vi "Command_ShootFromPose.vi"(0 "Startup":bool, 2 "Shooter_table":dbl[][](array[numeric]), 3 "Timeout":dbl) -> (11 "Reint":bool, 12 "turret_angle(deg)":dbl, 14 "Completed":bool, 15 "turret_state":T3=enum."No-Op", 16 "flywheel_state":T2, 17 "flywheel_speed(RPM)":dbl, 18 "cowl_state":T1=enum."No-Op", 19 "cowl_angle(deg)":dbl)   [LabVIEW 2020]
uses:
  Subsystems/Turret/Turret_States.ctl
  Subsystems/Flywheel/Flywheel_States.ctl
  Subsystems/Cowl/Cowl_States.ctl
  Auto Utilities/Command_Execution_State.ctl
  Globals/Sensor_Values.vi
  Systems/Shooter/Determiner/Shooter_Globals.vi
  Globals/Drive_Globals.vi
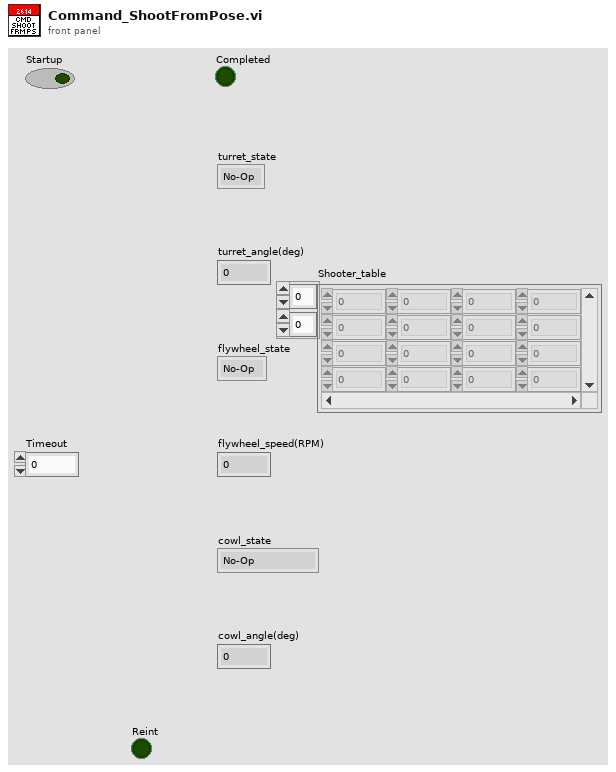
[diagram p1: front panel]
types:
  T1 = typedef "Cowl_States.ctl" = enum16{"Manual_%VBus", "GoToAngle", "No-Op", "GoToZero"}
  T2 = typedef "Flywheel_States.ctl" = enum16{"No-Op", "Percent_Voltage", "Speed_Control", "Speed_Control_Manual", "Command_SpinUp", "Command_SpinUpAuto"}
  T3 = typedef "Turret_States.ctl" = enum16{"Manual_Percent_Voltage", "Auto-Target", "Command_TurnToPosition", "Command_Auto_Target", "GoToZero", "No-Op", "Test_Position_Control", "Auto-Track"}
  T4 = typedef "Command_Execution_State.ctl" = enum16{"Initialize", "Execute", "Finish"}
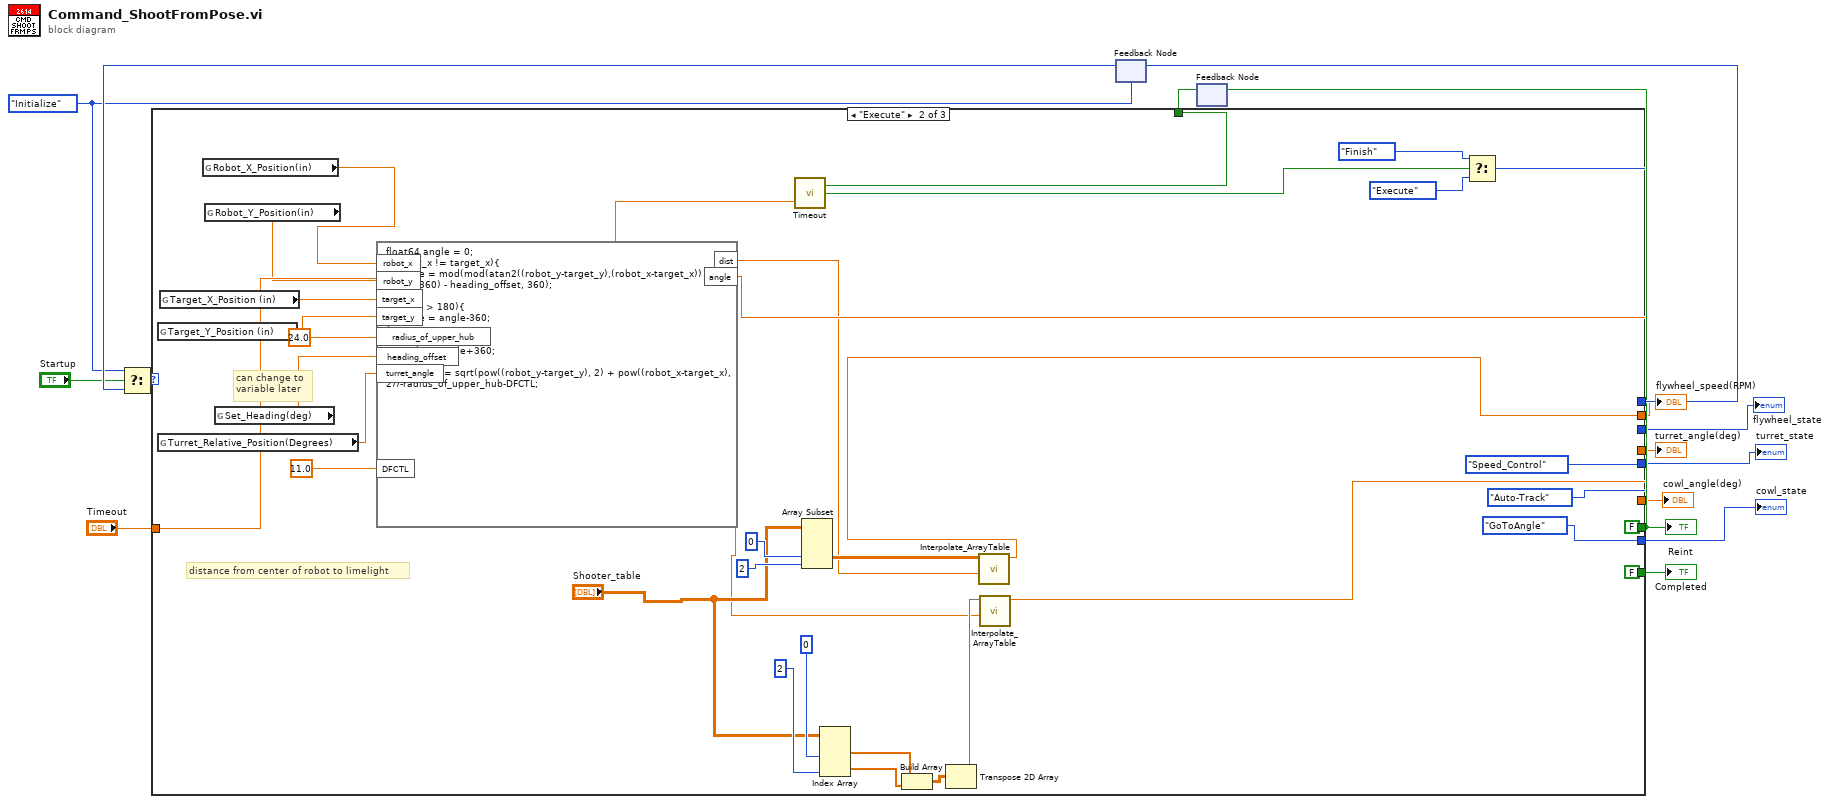
[diagram p0: block diagram]
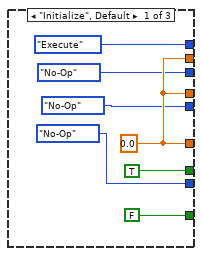
[diagram p2: hidden frame]
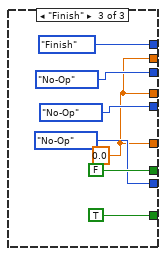
[diagram p3: hidden frame]
diagram:
  w10 = Command_Execution_State."Initialize" ("Play State")
  n1 = feedback #1(w10) -> (w13:T4)
  n2 = Select(t=w10, s="Startup", f=w13) -> (s? t:f=w15:T4)
  n3 = feedback #2() -> (w9:bool)  [unwired: 1 in]
  n4 = case shown="\"Execute\"" w15 {
    tunnel: [Command_Execution_State."Execute" ("Play State") w51 Command_Execution_State."Finish" ("Play State")] -> w14
    tunnel: [FALSE FALSE TRUE] -> w12
    tunnel: [TRUE FALSE FALSE] -> w7
    tunnel: w9 -> [_ w53 _]
    tunnel: "Timeout" -> [_ w52 _]
    tunnel: [w19 w35 w56] -> w6
    tunnel: [w19 w27 w56] -> w5
    tunnel: [w19 w36 w56] -> w4
    tunnel: [Flywheel_States."No-Op" ("flywheel_state") Flywheel_States."Speed_Control" ("flywheel_state") Flywheel_States."No-Op" ("flywheel_state")] -> w3
    tunnel: [Turret_States."No-Op" ("turret_state") Turret_States."Auto-Track" ("turret_state") Turret_States."No-Op" ("turret_state")] -> w2
    tunnel: [Cowl_States."No-Op" ("cowl_state") Cowl_States."GoToAngle" ("cowl_state") Cowl_States."No-Op" ("cowl_state")] -> w1
    frame "Initialize", Default {
      w19 = 0.0 ("cowl_angle(deg)")
    }
    frame "Execute" {
      # "distance from center of robot to limelight"
      # "can change to\nvariable later"
      n5 = global read "Shooter_Globals.vi" "Target_Y_Position (in)"() -> (w28:dbl)
      n6 = global read "Sensor_Values.vi" "Turret_Relative_Position(Degrees)"() -> (w23:dbl)
      n7 = global read "Shooter_Globals.vi" "Target_X_Position (in)"() -> (w29:dbl)
      n8 = global read "Sensor_Values.vi" "Robot_X_Position(in)"() -> (w32:dbl)
      n9 = global read "Sensor_Values.vi" "Robot_Y_Position(in)"() -> (w31:dbl)
      n10 = global read "Drive_Globals.vi" "Set_Heading(deg)"() -> (w25:dbl)
      n11 = formula code="float64 angle = 0;\nif(robot_x != target_x){\n    angle = mod(mod(atan2((robot_y-target_y),(robot_x-target_x)) * 180/pi,360) - heading_offset, 360);\n}\nif(angle > 180){\n    angle = angle-360;\n}\nif(angle < -180){\n    angle = angle+360;\n}\nfloat64 dist = sqrt(pow((robot_y-target_y), 2) + pow((robot_x-target_x), 2))-radius_of_upper_hub-DFCTL;"("robot_x"=w32, "robot_y"=w31, "target_x"=w29, "target_y"=w28, "radius_of_upper_hub"=24.0 ("input variable"), "heading_offset"=w25, "DFCTL"=11.0 ("input variable"), "turret_angle"=w23) -> ("dist"=w26:dbl, "angle"=w27:dbl)
      n12 = call "Timeout.vi"("Timeout"=w52, "Initialize"=w53) -> ("Timed Out?"=w48:bool)
      n13 = Array Subset(array="Shooter_table", index (col)=0 ("index"), length (col)=2 ("length")) -> (w44:dbl[][])  [unwired: 2 in]
      n14 = Index Array(array="Shooter_table", index (col) #1=0 ("index (row)"), index (col) #2=2 ("index (row)")) -> (element #1=w43:dbl[], element #2=w37:dbl[])  [unwired: 2 in]
      n15 = Build Array(w43, w37) -> (w41:dbl[][])
      n16 = Transpose 2D Array(2D array=w41) -> (transposed array=w40:dbl[][])
      n17 = call "Interpolate_ArrayTable.vi"("Desired_Distance"=w26, "array"=w44) -> ("RPM"=w36:dbl)  [unwired: 9 in]
      n18 = call "Interpolate_ArrayTable.vi"("Desired_Distance"=w26, "array"=w40) -> ("RPM"=w35:dbl)  [unwired: 9 in]
      n19 = Select(t=Command_Execution_State."Finish" ("Play State"), s=w48, f=Command_Execution_State."Execute" ("Play State")) -> (s? t:f=w51:T4)
    }
    frame "Finish" {
      w56 = 0.0 ("cowl_angle(deg)")
    }
  }
  "Completed" <- w12
  "Reint" <- w7
  "turret_state" <- w2
  "flywheel_state" <- w3
  "cowl_state" <- w1
  "turret_angle(deg)" <- w5
  "flywheel_speed(RPM)" <- w4
  "cowl_angle(deg)" <- w6
  n20 = feedback-in #1(w14) -> ()
  n21 = feedback-in #2(w7) -> ()
